vi "3D_Traverse_move_manual.vi"() -> ()   [LabVIEW 2011]
uses:
  Controls/Tunnel_Coordinates.ctl
  Controls/User_Specific_mode.ctl
  Trav_mode.ctl
panel:
  out "Current Pos":dbl[](array[numeric])
  in  "Work in Tunnel Coordinates":T1
  out "Current Traverse":string
  in  "Traverse":u16(ring) items=["Aero_Enclosure", "Aero_Sting", "Aero_Tunnel", "PIV_Traverse"]
  in  "stop":bool
  in  "Increment":dbl=10.0
  in  "Z-":bool
  in  "Z+":bool
  in  "Y+":bool
  in  "Y-":bool
  in  "X+":bool
  in  "X-":bool
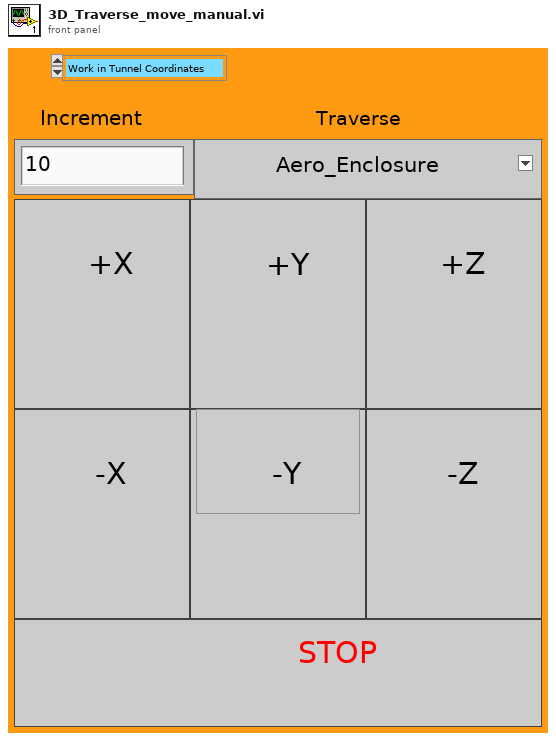
[diagram p1: front panel]
types:
  T1 = typedef "Tunnel_Coordinates.ctl" = enum16{"Work in Tunnel Coordinates", "Work in Model Coordinates"}
  T2 = typedef "User_Specific_mode.ctl" = enum16{"Check VI only", "Run VI"}
  T3 = typedef "Trav_mode.ctl" = enum16{"Move traverse", "Read traverse position", "Teach Position"}
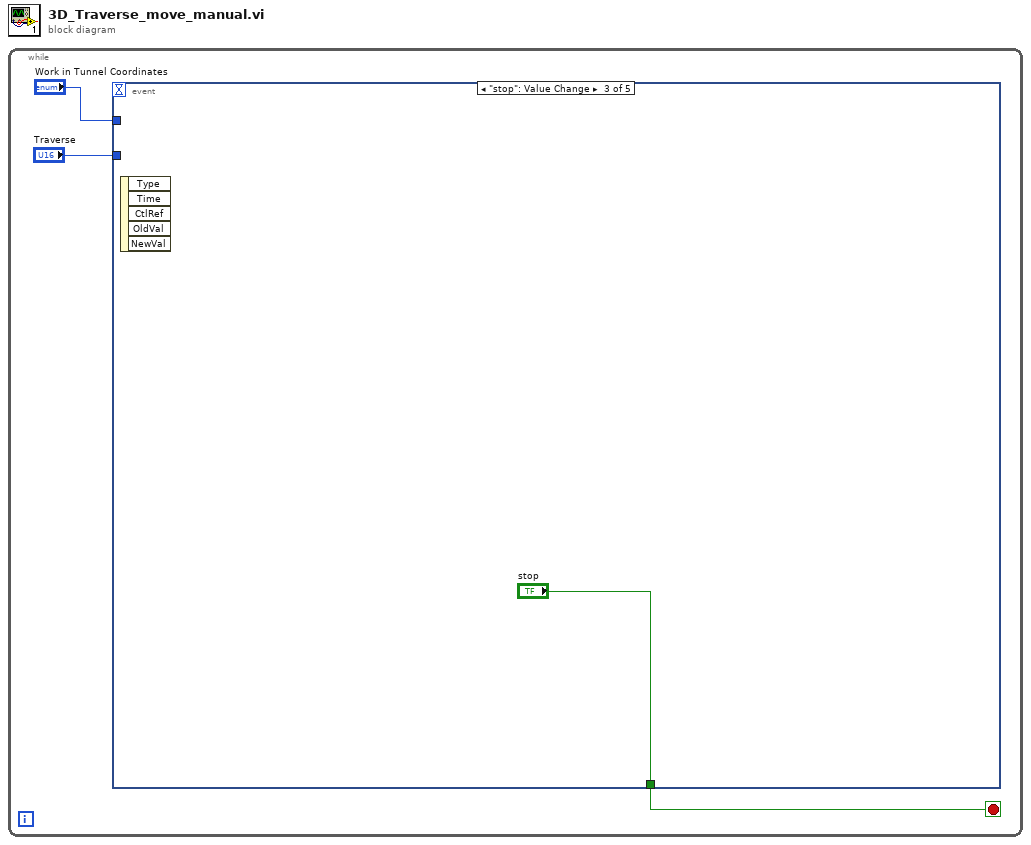
[diagram p0: block diagram]
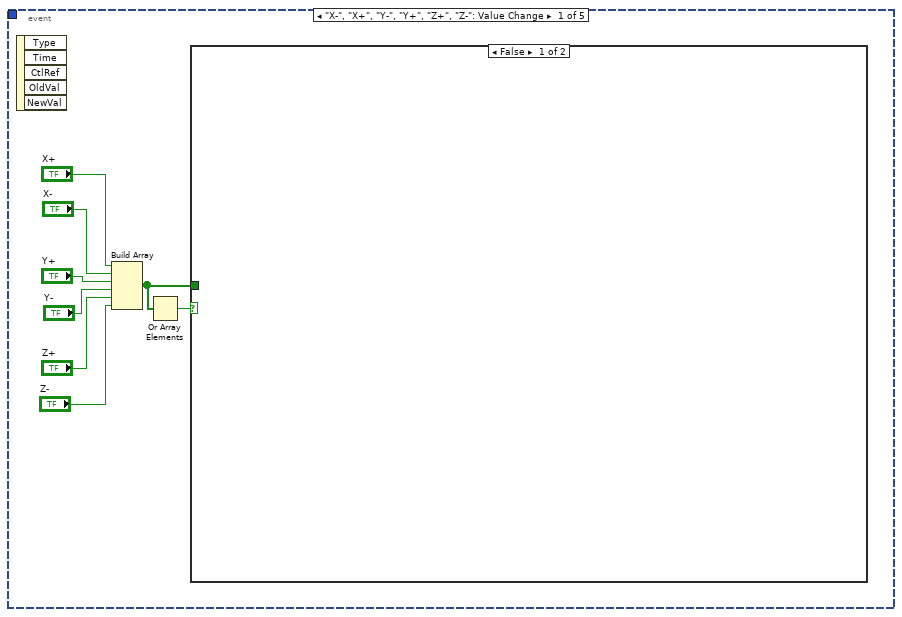
[diagram p2: hidden frame]
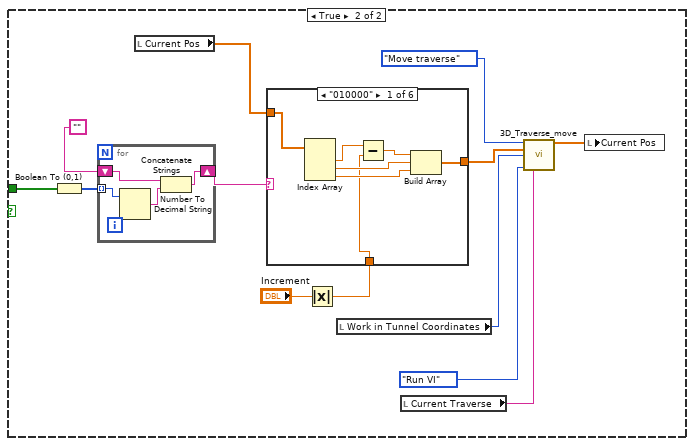
[diagram p3: hidden frame]
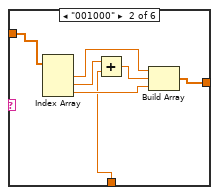
[diagram p4: hidden frame]
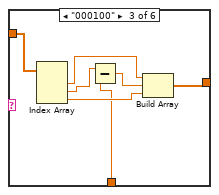
[diagram p5: hidden frame]
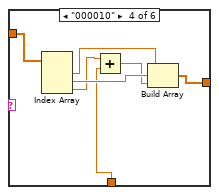
[diagram p6: hidden frame]
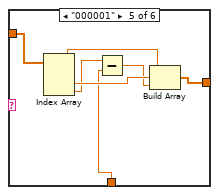
[diagram p7: hidden frame]
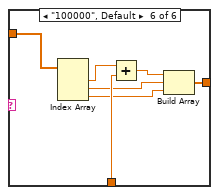
[diagram p8: hidden frame]
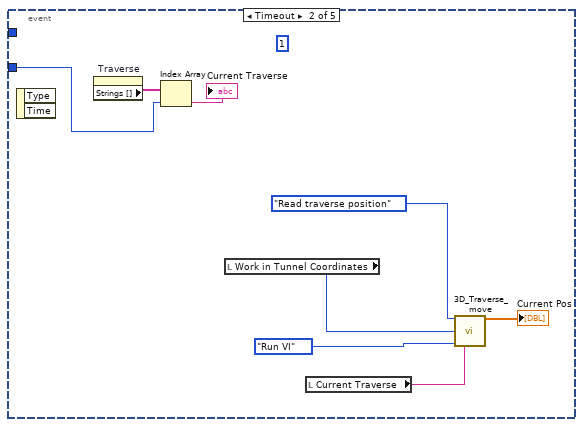
[diagram p9: hidden frame]
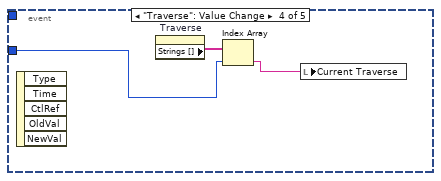
[diagram p10: hidden frame]
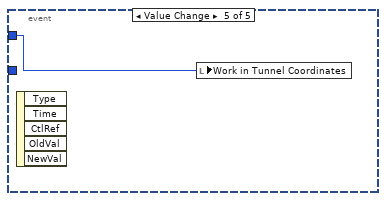
[diagram p11: hidden frame]
diagram:
  n1 = while {
    stop <- w3 stop-if-true
    n2 = event shown="[2] \"stop\": Value Change" {
      selector: _ -> [_ _ _ _ _]
      dyn-events: _ -> [_ _ _ _ _]
      timeout: _ -> [_ _ _ _ _]
      tunnel: [_ _ "stop" _ _] -> w3
      tunnel: "Traverse" -> [_ w71 _ w81 _]
      tunnel: "Work in Tunnel Coordinates" -> [_ _ _ _ w83]
      event "X-", "X+", "Y-", "Y+", "Z+", "Z-": Value Change {
        n3 = event-data() -> ()  [unwired: 1 in, 5 out]
        n4 = Build Array("X+", "X-", "Y+", "Y-", "Z+", "Z-") -> (w4:bool[])
        n5 = Or Array Elements(Boolean array=w4) -> (logical OR=w5:bool)
        n6 = case shown="False" w5 {
          tunnel: w4 -> [_ w12]
          frame False {
          }
          frame True {
            n7 = Boolean To (0,1)(Boolean=w12) -> (0, 1=w23:i16[])
            n8 = for {
              shift-right: [w27] -> w22
              shift-left: "" -> [w28]
              tunnel: w23 -> [w26] mode=indexing
              n9 = Number To Decimal String(number=w26) -> (decimal integer string=w25:string)  [unwired: 1 in]
              n10 = Concatenate Strings(w28, w25) -> (w27:string)
            }
            n11 = local read "Current Pos"() -> (w20:dbl[])
            n12 = Absolute Value(x="Increment") -> (abs(x)=w19:dbl)
            n13 = case shown="\"010000\"" w22 {
              tunnel: w20 -> [w29 w41 w45 w55 w62 w70]
              tunnel: w19 -> [w30 w40 w44 w51 w61 w68]
              tunnel: [w31 w36 w43 w50 w57 w64] -> w18
              frame "010000" {
                n14 = Index Array(array=w29) -> (element #1=w35:dbl, element #2=w33:dbl, element #3=w32:dbl)  [unwired: 3 in]
                n15 = Subtract(x=w35, y=w30) -> (x-y=w34:dbl)
                n16 = Build Array(w34, w33, w32) -> (w31:dbl[])
              }
              frame "001000" {
                n17 = Index Array(array=w41) -> (element #1=w38:dbl, element #2=w37:dbl, element #3=w42:dbl)  [unwired: 3 in]
                n18 = Add(x=w37, y=w40) -> (x+y=w39:dbl)
                n19 = Build Array(w38, w39, w42) -> (w36:dbl[])
              }
              frame "000100" {
                n20 = Index Array(array=w45) -> (element #1=w46:dbl, element #2=w48:dbl, element #3=w49:dbl)  [unwired: 3 in]
                n21 = Subtract(x=w48, y=w44) -> (x-y=w47:dbl)
                n22 = Build Array(w46, w47, w49) -> (w43:dbl[])
              }
              frame "000010" {
                n23 = Index Array(array=w55) -> (element #1=w52:dbl, element #2=w56:dbl, element #3=w54:dbl)  [unwired: 3 in]
                n24 = Add(x=w54, y=w51) -> (x+y=w53:dbl)
                n25 = Build Array(w52, w56, w53) -> (w50:dbl[])
              }
              frame "000001" {
                n26 = Index Array(array=w62) -> (element #1=w58:dbl, element #2=w63:dbl, element #3=w60:dbl)  [unwired: 3 in]
                n27 = Subtract(x=w60, y=w61) -> (x-y=w59:dbl)
                n28 = Build Array(w58, w63, w59) -> (w57:dbl[])
              }
              frame "100000", Default {
                n29 = Index Array(array=w70) -> (element #1=w69:dbl, element #2=w66:dbl, element #3=w65:dbl)  [unwired: 3 in]
                n30 = Add(x=w69, y=w68) -> (x+y=w67:dbl)
                n31 = Build Array(w67, w66, w65) -> (w64:dbl[])
              }
            }
            n32 = local read "Work in Tunnel Coordinates"() -> (w15:T1)
            n33 = local read "Current Traverse"() -> (w13:string)
            n34 = call "3D_Traverse_move.vi"("Mode"=Trav_mode."Move traverse", "Position"=w18, "Work in Tunnel Coordinates"=w15, "Simulate/Run"=User_Specific_mode."Run VI", "Traverse name"=w13) -> ("Trav Position achieved"=w17:dbl[])  [unwired: 8 in, 2 out]
            n35 = local write "Current Pos"(w17) -> ()
          }
        }
      }
      event Timeout {
        (unwired) 1
        n36 = event-data() -> ()  [unwired: 1 in, 2 out]
        n37 = property on="Traverse" class="Ring (strict)"() -> ("Strings []"=w72:string[])  [unwired: 2 in, 2 out]
        n38 = Index Array(array=w72, index=w71) -> (element=→"Current Traverse":string)
        n39 = local read "Work in Tunnel Coordinates"() -> (w74:T1)
        n40 = local read "Current Traverse"() -> (w75:string)
        n41 = call "3D_Traverse_move.vi"("Mode"=Trav_mode."Read traverse position" ("Mode 2"), "Work in Tunnel Coordinates"=w74, "Simulate/Run"=User_Specific_mode."Run VI" ("Simulate/Run 2"), "Traverse name"=w75) -> ("Trav Position achieved"=→"Current Pos":dbl[])  [unwired: 9 in, 2 out]
      }
      event "stop": Value Change {
        n42 = event-data() -> ()  [unwired: 1 in, 5 out]
      }
      event "Traverse": Value Change {
        n43 = event-data() -> ()  [unwired: 1 in, 5 out]
        n44 = property on="Traverse" class="Ring (strict)"() -> ("Strings []"=w82:string[])  [unwired: 2 in, 2 out]
        n45 = Index Array(array=w82, index=w81) -> (element=w80:string)
        n46 = local write "Current Traverse"(w80) -> ()
      }
      event Value Change {
        n47 = event-data() -> ()  [unwired: 1 in, 5 out]
        n48 = local write "Work in Tunnel Coordinates"(w83) -> ()
      }
    }
  }
